vi "done initial writing.vi"() -> ()   [LabVIEW 2022 SP3]
panel:
  out "done initial writing":bool
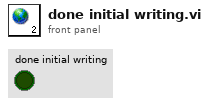
[diagram p1: front panel]
diagram:
